vi "get waveform.vi"(6 "warning":bool=TRUE, 7 "file path":path, 8 "phase":i32, 9 "f":dbl=0.0078125 format="%.4e", 10 "amplitude":dbl format="%.2f", 11 "samples":i32=128) -> (0 "discontinuities":bool, 3 "waveform":sgl[](array[numeric]) format="%.2f", 5 "new file path":path)   [LabVIEW 2010]
uses:
  <vilib>/Utility/file.llb/Read From Spreadsheet File (DBL).vi
  <vilib>/Analysis/NI_AALBase.lvlib
  <vilib>/Analysis/NI_AALPro.lvlib
panel:
  # "ticks"
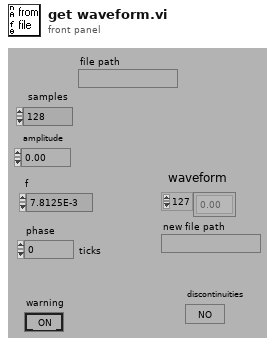
[diagram p1: front panel]
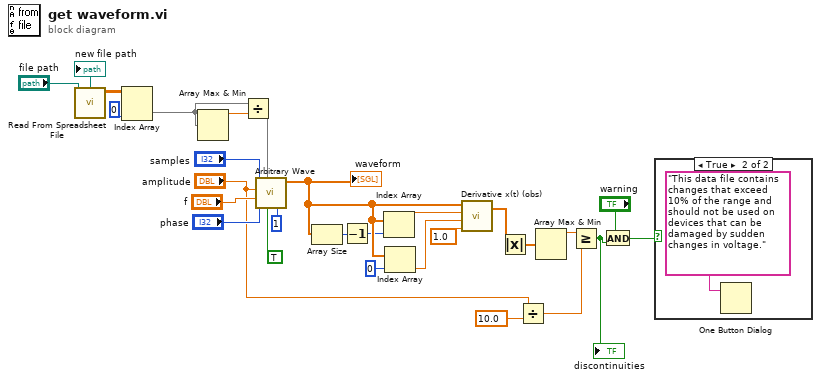
[diagram p0: block diagram]
diagram:
  n1 = call-poly <vilib>:"Read From Spreadsheet File.vi"("file path (dialog if empty)"="file path") -> ("all rows"=w28:dbl[][], "new file path (Not A Path if cancelled)"=→"new file path":path)  [unwired: 6 in, 3 out]
  n2 = Index Array(array=w28, index (col)=0) -> (element=w19:dbl[])  [unwired: 1 in]
  n3 = Array Max & Min(array=w19) -> (max value=w24:dbl)  [unwired: 3 out]
  n4 = Divide(x=w19, y=w24) -> (x/y=w18:dbl[])
  n5 = call <vilib>:"Arbitrary Wave.vi"("interpolation"=1, "reset phase"=TRUE, "Wave Table"=w18, "phase in"="phase", "frequency"="f", "amplitude"="amplitude", "samples"="samples") -> ("arbitrary wave"=w17:dbl[])  [unwired: 2 out]
  "waveform" <- w17
  n6 = Array Size(array=w17) -> (size(s)=w15:i32)
  n7 = Decrement(x=w15) -> (x-1=w14:i32)
  n8 = Index Array(array=w17, index=w14) -> (element=w13:dbl)
  n9 = Index Array(array=w17, index=0) -> (element=w12:dbl)
  n10 = call <vilib>:"Derivative x(t) (obs).vi"("dt"=1.0, "final condition"=w12, "initial condition"=w13, "X"=w17) -> ("dX/dt"=w9:dbl[])  [unwired: 1 out]
  n11 = Absolute Value(x=w9) -> (abs(x)=w8:dbl[])
  n12 = Divide(x="amplitude", y=10.0) -> (x/y=w6:dbl)
  n13 = Array Max & Min(array=w8) -> (max value=w7:dbl)  [unwired: 3 out]
  n14 = Greater Or Equal?(x=w7, y=w6) -> (x >= y?=w1:bool)
  "discontinuities" <- w1
  n15 = And(x="warning", y=w1) -> (x .and. y?=w3:bool)
  n16 = case shown="True" w3 {
    frame False {
    }
    frame True {
      n17 = One Button Dialog(message="This data file contains changes that exceed 10% of the range and should not be used on devices that can be damaged by sudden changes in voltage.") -> ()  [unwired: 1 in, 1 out]
    }
  }
